vi "NI VeriStand - Get Custom Device Waveform Data.vi"(8 "error in (no error)":errorcluster, 11 "Waveform Ref in":T3 format="%.0x") -> (0 "error out":errorcluster, 1 "Waveform":T1, 2 "Waveform Name":string, 3 "Waveform Ref out":T3 format="%.0x", 4 "Found":bool, 5 "GUID":string)   [LabVIEW 2020, in "Custom Device API.lvlib"]
doc: "Returns information about the waveform item specified by <B>Waveform Ref in</B>."
uses:
  <vilib>/NI VeriStand/Custom Device API/Custom Device API.lvlib
  <vilib>/NI VeriStand/Custom Device API/Custom Device Item Ref.ctl
  <vilib>/NI VeriStand/Custom Device API/Custom Device Waveform.ctl
  <vilib>/NI VeriStand/Custom Device API/Custom Device Waveform DataType.ctl
  a7ed12f7-5412-47db-9470-1187f47309fb.vi
  <vilib>/NI VeriStand/Custom Device API/Custom Device Offline Path.vi
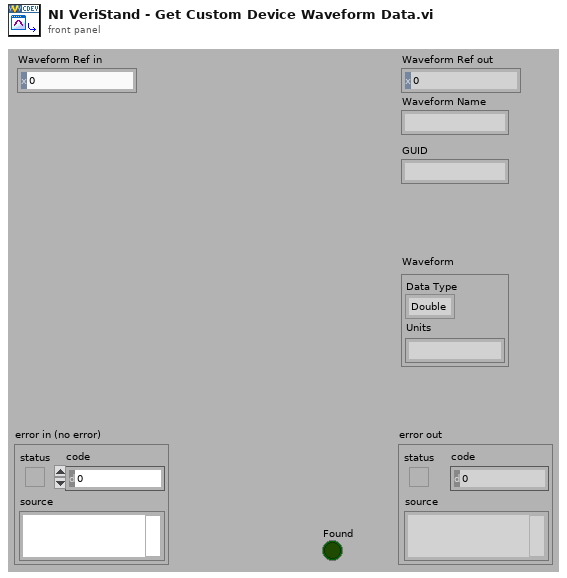
[diagram p1: front panel]
types:
  T1 = typedef "Custom Device API.lvlib/Custom Device Waveform.ctl" = cluster{"Data Type":T2, "Units":string}
  T2 = typedef "Custom Device API.lvlib/Custom Device Waveform DataType.ctl" = enum16{"Double", "Complex Double"}
  T3 = typedef "Custom Device API.lvlib/Custom Device Item Ref.ctl" = u64
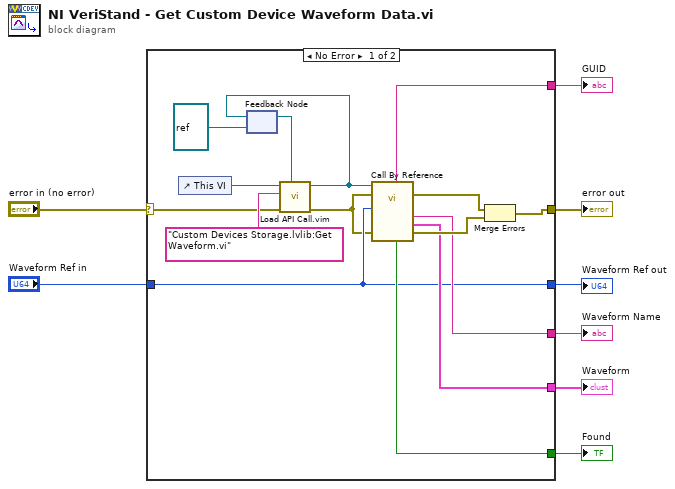
[diagram p0: block diagram]
diagram:
  n1 = case shown="No Error" "error in (no error)" {
    selector: "error in (no error)" -> [w10 w25]
    tunnel: "Waveform Ref in" -> [w17 w24]
    tunnel: [w17 w24] -> w7
    tunnel: [w22 _] -> w6
    tunnel: [w21 _] -> w5
    tunnel: [w20 w25] -> w4
    tunnel: [w19 _] -> w3
    tunnel: [w18 _] -> w2
    frame No Error {
      n2 = control-ref of="This VI"() -> (w15:refnum<vi>)
      n3 = feedback #1(refnum<vi> refnum ("type specifier VI Refnum (for type only)")) -> (w16:refnum<vi>)
      n4 = call "Load API Call.vim"("VI reference in"=w16, "error in (no error)"=w10, "VI qualified name"="Custom Devices Storage.lvlib:Get Waveform.vi", "Caller VI ref"=w15) -> ("error out"=w12:errorcluster, "VI reference"=w13:refnum<vi>)  [unwired: 6 in]
      n5 = feedback-in #1(w13) -> ()
      n6 = call-by-ref "?"(reference=w13, error in=w12, 8:"error in (no error)"=w12, "Waveform Ref in"=w17) -> (error out=w9:errorcluster, 0:"error out"=w23:errorcluster, "Waveform"=w19:T1, "Waveform Name"=w22:string, "Found"=w21:bool, "GUID"=w18:string)  [unwired: 4 in, 2 out]
      n7 = Merge Errors(w9, w23) -> (w20:errorcluster)
    }
    frame Error {
    }
  }
  "Waveform Ref out" <- w7
  "error out" <- w4
  "Waveform" <- w3
  "Found" <- w5
  "GUID" <- w2
  "Waveform Name" <- w6
